vi "Multimeter.vi"(10 "GPIB Address":string, 11 "error in":errorcluster) -> (0 "error out":errorcluster, 3 "Voltage":dbl)   [LabVIEW 2017, in "LD Reading.lvclass"]
uses:
  LD Reading.lvclass
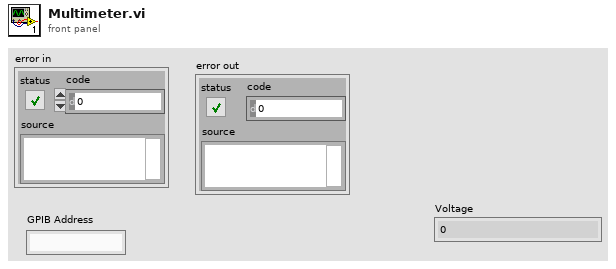
[diagram p1: front panel]
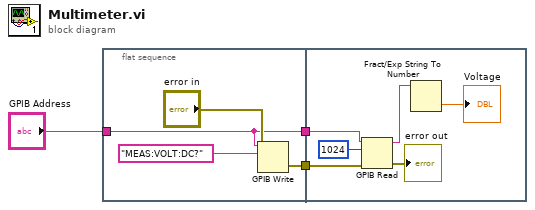
[diagram p0: block diagram]
diagram:
  n1 = flat-sequence {
    tunnel: [w6] -> w3
    tunnel: "GPIB Address" -> [w4]
    tunnel: [w4] -> w2
    tunnel: w3 -> [w13]
    tunnel: w2 -> [w8]
    frame #0 {
      n2 = GPIB Write(0:w4, 1:"MEAS:VOLT:DC?" ("data"), 3:"error in") -> (6:w6:errorcluster)  [unwired: 2 in, 1 out]
    }
    frame #1 {
      n3 = GPIB Read(0:w8, 1:1024 ("byte count"), 3:w13) -> (5:w11:string, 7:→"error out":errorcluster)  [unwired: 2 in, 1 out]
      n4 = Fract/Exp String To Number(string=w11) -> (number=→"Voltage":dbl)  [unwired: 3 in, 1 out]
    }
  }
